vi "Test 7z.bat.vi"() -> ()   [LabVIEW 2016]
uses:
  PostBuildSupport (2013).lvclass
panel:
  in  "Product Name":string
  in  "Package Source Folder":path
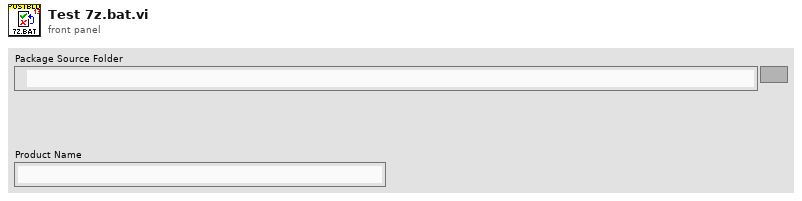
[diagram p1: front panel]
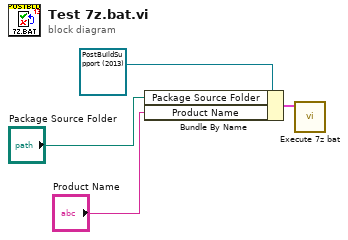
[diagram p0: block diagram]
diagram:
  n1 = Bundle By Name(cluster=refnum<class "PostBuildSupport (2013).lvclass"> refnum ("PostBuildSupport in"), "Package Source Folder"="Package Source Folder", "Product Name"="Product Name") -> (w1:cluster{})
  n2 = call "Execute 7z bat.vi"("PostBuildSupport in"=w1) -> ()  [unwired: 9 in, 2 out]
